vi "String To 1D String Array.vi"(11 "String":string) -> (3 "Array[]":string[](array[string]))   [LabVIEW 2023, in "SLL Environment Variable.lvlib"]
doc: "Convert string to 1D string array."
uses:
  SLL Environment Variable.lvlib
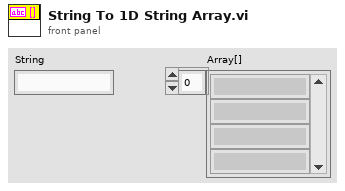
[diagram p1: front panel]
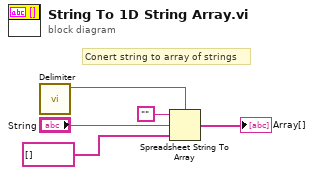
[diagram p0: block diagram]
diagram:
  # "Conert string to array of strings"
  n1 = call "Delimiter.vi"() -> ("Delimiter"=w1:string)  [unwired: 11 in]
  n2 = Spreadsheet String To Array(delimiter (Tab)=w1, format string="", spreadsheet string="String", array type (2D Dbl)=string[] []) -> (array=→"Array[]":string[])
